vi "Abs.vi"(11 "A":dbl) -> (3 "C":dbl)   [LabVIEW 2018]
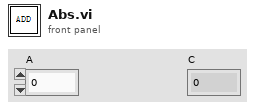
[diagram p1: front panel]
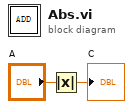
[diagram p0: block diagram]
diagram:
  n1 = Absolute Value(x="A") -> (abs(x)=→"C":dbl)
